vi "写入量程参数.vi"(8 "error in (no error)":errorcluster, 10 "自动测试量程配置":T2={"水样测试量程模式"=enum."H", "标样核查量程模式"=enum."H", "零点核查量程模式"=enum."H", "跨度核查量程模式"=enum."H", "空白测试量程模式"=enum."H", "平行样测试量程模式"=enum."H", "加标回收量程模式"=enum."H", "空白校准量程模式"=enum."H", "标样校准量程模式"=enum."H"}, 11 "MB session in":refnum<class "MB_Master.lvclass">) -> (0 "error out":errorcluster, 3 "MB session out":refnum<class "MB_Master.lvclass">)   [LabVIEW 2016, in "斯坦道CODMn新电路板.lvlib"]
uses:
  <vilib>/Plasmionique/MB Master/MB_Master/MB_Master.lvclass
  <vilib>/Plasmionique/MB Master/MB_Master_Serial/MB_Master_Serial.lvclass
  C:/Program Files (x86)/National Instruments/LabVIEW 2016/vi.lib/Plasmionique/MB Master/MB_Master/MB_Master.lvclass
  <vilib>/Plasmionique/MB Master/MB Master.lvlib
panel:
  in  "VISA Resource":refnum<visa-resource-name>
  in  "引用选择":enum16{"MB引用", "自建引用"}(ring)
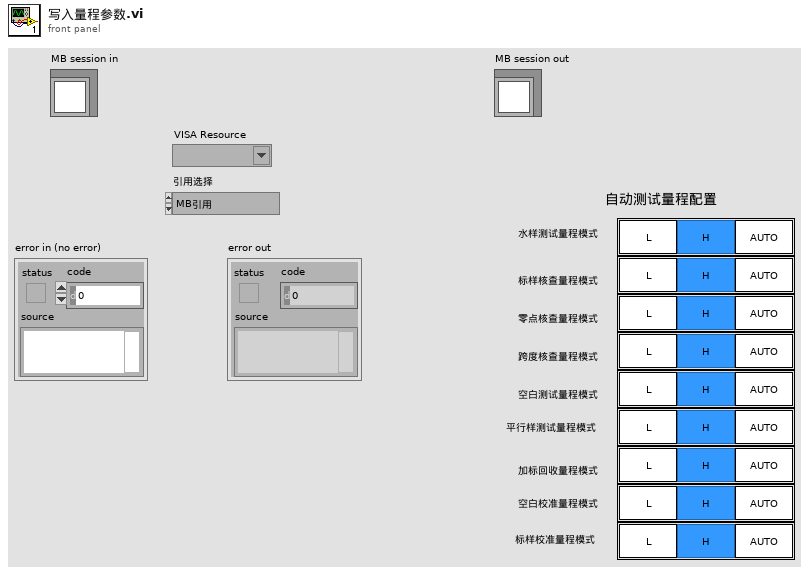
[diagram p1: front panel]
types:
  T1 = typedef "量程选择控件.ctl" = enum32{"L", "H", "AUTO"}
  T2 = cluster{"水样测试量程模式":T1, "标样核查量程模式":T1, "零点核查量程模式":T1, "跨度核查量程模式":T1, "空白测试量程模式":T1, "平行样测试量程模式":T1, "加标回收量程模式":T1, "空白校准量程模式":T1, "标样校准量程模式":T1}
  T3 = cluster{"baud rate (bps)":u32, "stop bits":u16, "parity":u16, "flow control":u16, "timeout":u32, "retries":i32}
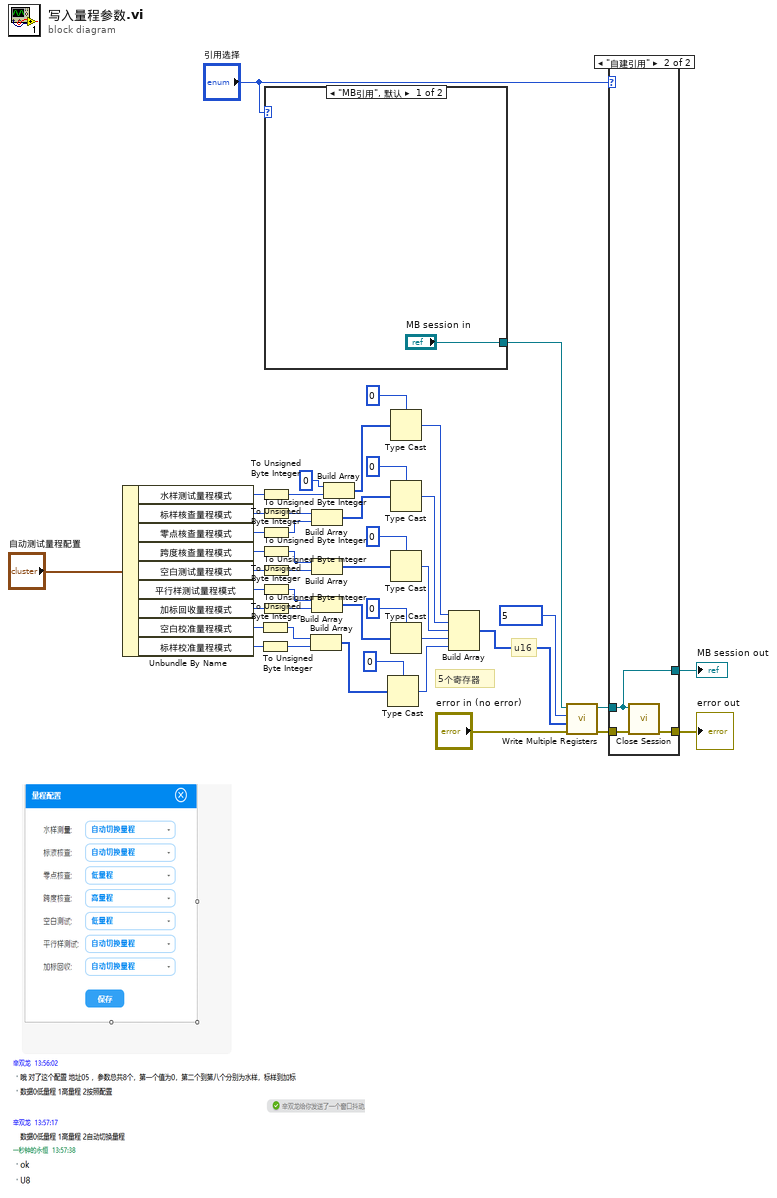
[diagram p0: block diagram]
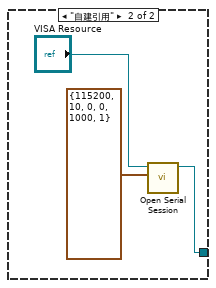
[diagram p3: hidden frame]
diagram:
  # "5个寄存器"
  # "u16"
  n1 = Unbundle By Name("自动测试量程配置") -> ("水样测试量程模式"=w21:T1, "标样核查量程模式"=w19:T1, "零点核查量程模式"=w17:T1, "跨度核查量程模式"=w15:T1, "空白测试量程模式"=w14:T1, "平行样测试量程模式"=w12:T1, "加标回收量程模式"=w11:T1, "空白校准量程模式"=w5:T1, "标样校准量程模式"=w4:T1)
  n2 = To Unsigned Byte Integer(number=w5) -> (unsigned 8bit integer=w6:u8)
  n3 = To Unsigned Byte Integer(number=w4) -> (unsigned 8bit integer=w7:u8)
  n4 = To Unsigned Byte Integer(number=w21) -> (unsigned 8bit integer=w20:u8)
  n5 = To Unsigned Byte Integer(number=w19) -> (unsigned 8bit integer=w18:u8)
  n6 = To Unsigned Byte Integer(number=w17) -> (unsigned 8bit integer=w16:u8)
  n7 = To Unsigned Byte Integer(number=w15) -> (unsigned 8bit integer=w9:u8)
  n8 = To Unsigned Byte Integer(number=w14) -> (unsigned 8bit integer=w8:u8)
  n9 = To Unsigned Byte Integer(number=w12) -> (unsigned 8bit integer=w13:u8)
  n10 = To Unsigned Byte Integer(number=w11) -> (unsigned 8bit integer=w10:u8)
  n11 = case shown="\"MB引用\", 默认" "引用选择" {
    tunnel: ["MB session in" w48] -> w42
    frame "MB引用", Default {
    }
    frame "自建引用" {
      n12 = call <vilib>:"Open Serial Session.vi"("Serial Config"=T3 {"baud rate (bps)"=115200, "stop bits"=10, "parity"=0, "flow control"=0, "timeout"=1000, "retries"=1}, "VISA Resource"="VISA Resource") -> ("MB_Serial session"=w48:refnum<class "MB_Master_Serial.lvclass">)  [unwired: 8 in, 1 out]
    }
  }
  n13 = Build Array(w6, w7) -> (w2:u8[])
  n14 = Build Array(w18, w16) -> (w34:u8[])
  n15 = Build Array(w9, w8) -> (w24:u8[])
  n16 = Build Array(w13, w10) -> (w29:u8[])
  n17 = Build Array(u8 0, w20) -> (w35:u8[])
  n18 = Type Cast(type=u16 0, x=w2) -> (*(type *) &x=w1:u16)
  n19 = Type Cast(type=u16 0, x=w35) -> (*(type *) &x=w31:u16)
  n20 = Type Cast(type=u16 0, x=w34) -> (*(type *) &x=w30:u16)
  n21 = Type Cast(type=u16 0, x=w24) -> (*(type *) &x=w23:u16)
  n22 = Type Cast(type=u16 0, x=w29) -> (*(type *) &x=w22:u16)
  n23 = Build Array(w31, w30, w23, w22, w1) -> (w32:u16[])
  n24 = call <vilib>:"Write Multiple Registers.vi"("error in (no error)"="error in (no error)", "values"=w32, "starting address"=u16 5, "MB session in"=w42) -> ("error out"=w39:errorcluster, "MB session out"=w41:refnum<class "MB_Master.lvclass">)  [unwired: 6 in]
  n25 = case shown="\"自建引用\"" "引用选择" {
    tunnel: w41 -> [w49 w51]
    tunnel: w39 -> [w50 w53]
    tunnel: [w50 w52] -> w38
    tunnel: [w49 w51] -> w37
    frame "MB引用", Default {
    }
    frame "自建引用" {
      n26 = call-dynamic "Close Session.vi"("error in (no error)"=w53, "MB session in"=w51) -> ("error out"=w52:errorcluster)  [unwired: 9 in]
    }
  }
  "MB session out" <- w37
  "error out" <- w38
